vi "IB_1200_1300_Project_SoftDep.vi"(7 "action":T3, 8 "error in (no error)":errorcluster, 9 "index in":string, 10 "dataSource in":T2, 11 "buildObject":T1) -> (0 "error out":errorcluster, 1 "index out":string, 2 "dataSource out":T2, 3 "buildObject out":T1)   [LabVIEW 2020]
doc: "Reads and writes the data to the object property bag."
uses:
  <resource>/Framework/Providers/API/ItemRef.ctl
  <vilib>/AppBuilder/IB_RW_Project/IB_RW_Project_PropBag_Action.ctl
  <vilib>/AppBuilder/IB_RW_Project/Compatibility/IB_2012_2013_Project_SoftDep_Data.ctl
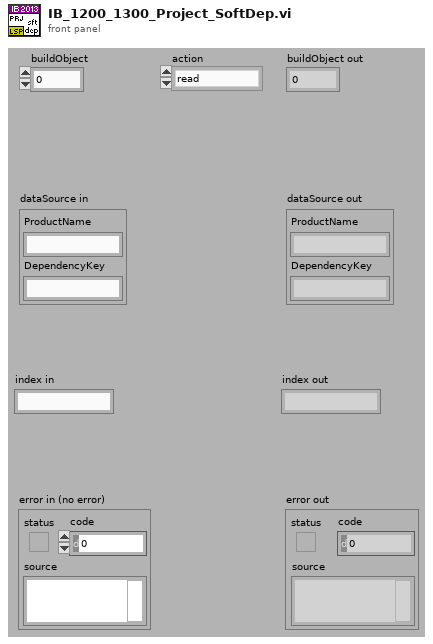
[diagram p1: front panel]
types:
  T1 = typedef "ItemRef.ctl" = u64
  T2 = typedef "IB_2012_2013_Project_SoftDep_Data.ctl" = cluster{"ProductName":string, "DependencyKey":string}
  T3 = typedef "IB_RW_Project_PropBag_Action.ctl" = enum16{"read", "write", "clear", "readPrevious", "writePrevious", "clearPrevious"}
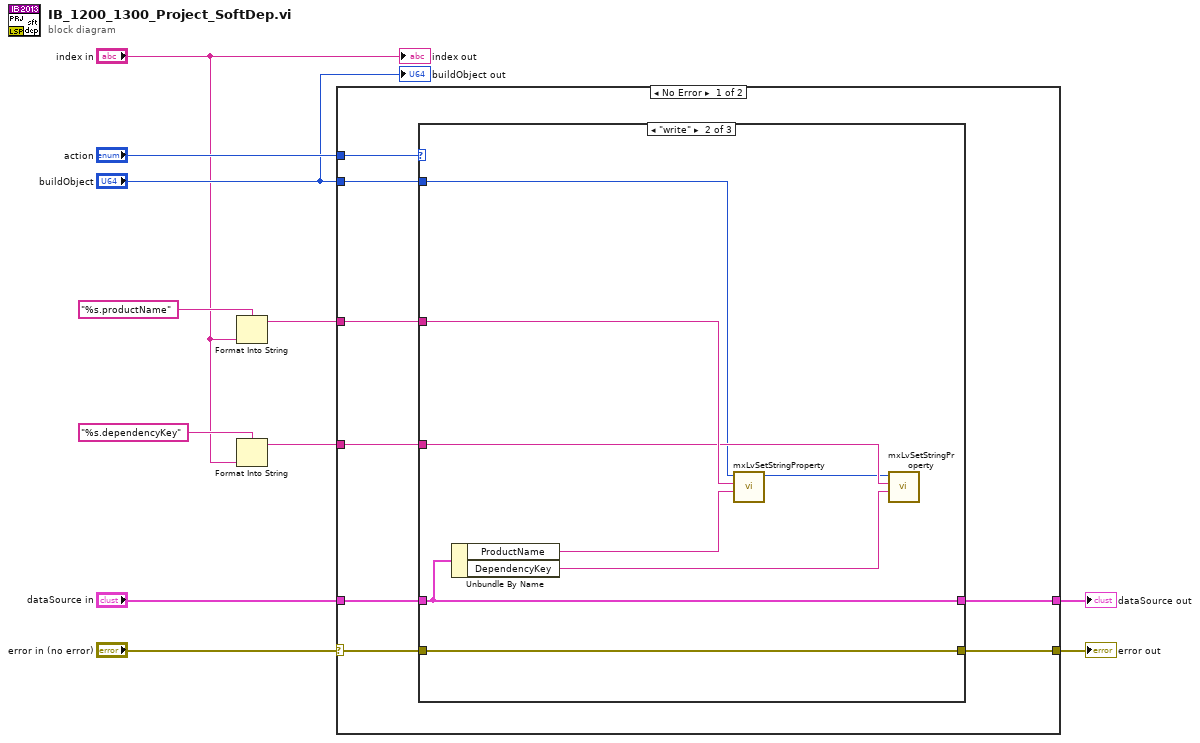
[diagram p0: block diagram]
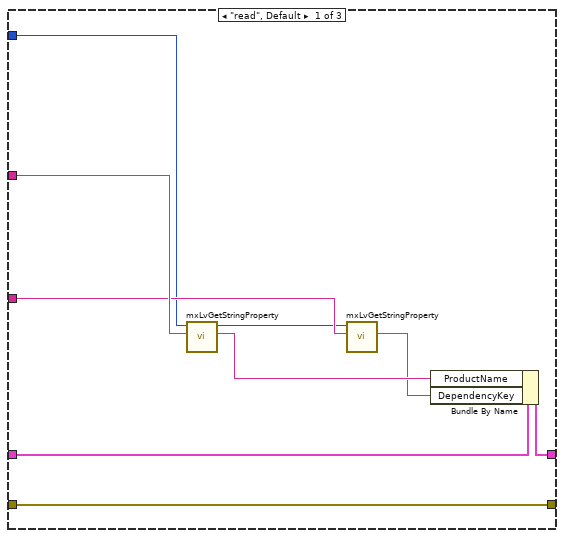
[diagram p2: hidden frame]
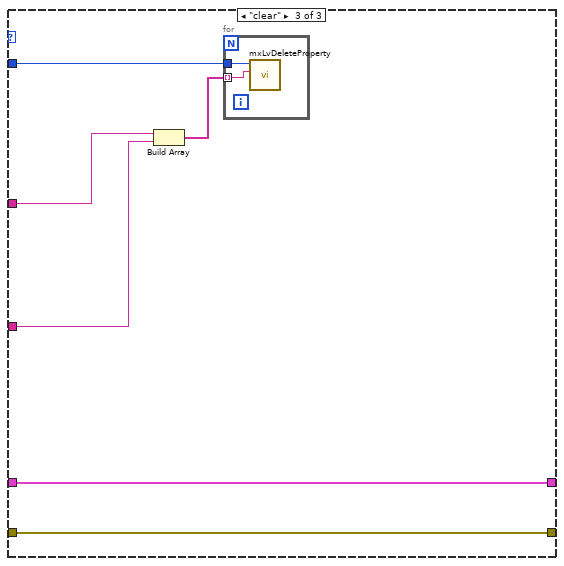
[diagram p3: hidden frame]
diagram:
  n1 = Format Into String(format string="%s.productName", "index in") -> (resulting string=w6:string)  [unwired: 2 in, 1 out]
  n2 = Format Into String(format string="%s.dependencyKey", "index in") -> (resulting string=w2:string)  [unwired: 2 in, 1 out]
  n3 = case shown="No Error" "error in (no error)" {
    selector: "error in (no error)" -> [w15 w45]
    tunnel: "action" -> [w19 _]
    tunnel: "dataSource in" -> [w18 w46]
    tunnel: [w17 w46] -> w9
    tunnel: "buildObject" -> [w13 _]
    tunnel: w6 -> [w16 _]
    tunnel: [w12 w45] -> w5
    tunnel: w2 -> [w14 _]
    frame No Error {
      n4 = case shown="\"write\"" w19 {
        tunnel: w13 -> [w21 w30 w38]
        tunnel: w18 -> [w28 w36 w42]
        tunnel: [w27 w36 w42] -> w17
        tunnel: w16 -> [w26 w33 w40]
        tunnel: [w25 w35 w39] -> w12
        tunnel: w15 -> [w25 w35 w39]
        tunnel: w14 -> [w23 w32 w37]
        frame "read", Default {
          n5 = call <resource>:"mxLvGetStringProperty.vi"("Tag"=w26, "Item"=w21) -> ("Value"=w24:string, "Item"=w20:T1)  [unwired: 1 in, 7 out]
          n6 = call <resource>:"mxLvGetStringProperty.vi"("Tag"=w23, "Item"=w20) -> ("Value"=w22:string)  [unwired: 1 in, 8 out]
          n7 = Bundle By Name(cluster=w28, "ProductName"=w24, "DependencyKey"=w22) -> (w27:T2)
        }
        frame "write" {
          n8 = Unbundle By Name(w36) -> ("ProductName"=w34:string, "DependencyKey"=w31:string)
          n9 = call <resource>:"mxLvSetStringProperty.vi"("Value (\"\")"=w34, "Tag"=w33, "Item"=w30) -> ("Item"=w29:T1)  [unwired: 2 in, 6 out]
          n10 = call <resource>:"mxLvSetStringProperty.vi"("Value (\"\")"=w31, "Tag"=w32, "Item"=w29) -> ()  [unwired: 2 in, 7 out]
        }
        frame "clear" {
          n11 = Build Array(w40, w37) -> (w41:string[])
          n12 = for {
            tunnel: w41 -> [w44] mode=indexing
            tunnel: w38 -> [w43]
            n13 = call <resource>:"mxLvDeleteProperty.vi"("Tag"=w44, "Item"=w43) -> ()  [unwired: 1 in, 9 out]
          }
        }
      }
    }
    frame Error {
    }
  }
  "error out" <- w5
  "dataSource out" <- w9
  "buildObject out" <- "buildObject"
  "index out" <- "index in"
